vi "To Serial Form.vi"(6 "Serial Version":T1, 10 "Serializer in":refnum<class "Serializer.lvclass">, 11 "CRDS Cell in":refnum<class "CRDS Cell.lvclass">) -> (0 "error out":errorcluster, 2 "Serializer out":refnum<class "Serializer.lvclass">, 3 "CRDS Cell out":refnum<class "CRDS Cell.lvclass">)   [LabVIEW 2012, in "CRDS Cell.lvclass"]
uses:
  CRDS Cell.lvclass
  <userlib>/Serialization/Serializer/Serializer.lvclass
  <userlib>/Serialization/Serialization Common/Serial Version.ctl
  <userlib>/Serialization/Serializable/Serializable.lvclass
  CRDS Cell.lvclass/CRDS Cell.ctl
  Get Tau Method.ctl
  <userlib>/Serialization/Serializer/Serializer.lvclass/Serializer.ctl
  <userlib>/Serialization/Formatter/Formatter.lvclass/Formatter.ctl
  <userlib>/Serialization/Serializable/Insert Double.vi
  <userlib>/Serialization/Serializable/Insert Single.vi
  <userlib>/Serialization/Serializable/Insert Int08.vi
  <userlib>/Serialization/Serializable/Insert Boolean.vi
  <userlib>/Serialization/Serializable/Insert UInt08.vi
  <userlib>/Serialization/Serializer/Insert Double.vi
  <userlib>/Serialization/Serializer/Insert Single.vi
  <userlib>/Serialization/Serializer/Insert Int08.vi
  <userlib>/Serialization/Serializer/Insert Boolean.vi
  <userlib>/Serialization/Serializer/Insert UInt08.vi
  <userlib>/Serialization/Formatter/Read Include all fields.vi
  <userlib>/Serialization/Serialization Common/Serialization Common.lvlib
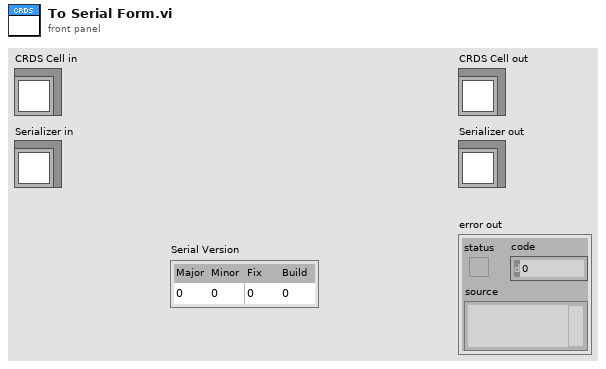
[diagram p1: front panel]
types:
  T1 = typedef "Serialization Common.lvlib/Serial Version.ctl" = cluster{"Major":u16, "Minor":u16, "Fix":u16, "Build":u16}
  T2 = typedef "Get Tau Method.ctl" = enum8{"DFT-1", "DFT-5", "LRS"}
  T3 = cluster{"inSeriesPos":u8, "numInBank":u8, "totNum":u8}
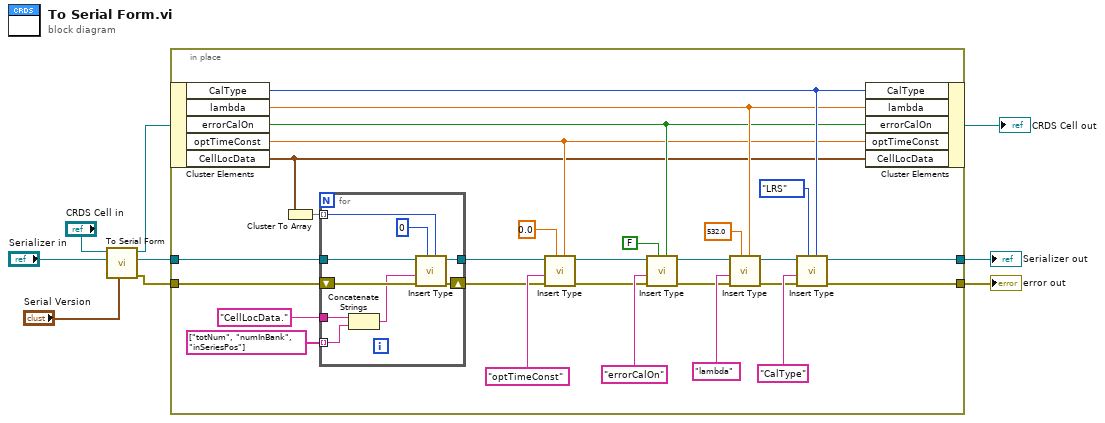
[diagram p0: block diagram]
diagram:
  n1 = call-parent "To Serial Form.vi"("Serial Version"="Serial Version", "Serializer in"="Serializer in", "Serializable in"="CRDS Cell in") -> ("error out"=w2:errorcluster, "Serializer out"=w5:refnum<class "Serializer.lvclass">, "Serializable out"=w6:refnum<class "CRDS Cell.lvclass">)  [unwired: 6 in]
  n2 = in-place {
    in-place-border: w5 -> [w11]
    in-place-border: [w29] -> w3
    in-place-border: w2 -> [w10]
    in-place-border: [w24] -> w1
    n3 = in-place-cluster #1(w6) -> ("CalType"=w19:T2, "lambda"=w18:dbl, "errorCalOn"=w17:bool, "optTimeConst"=w16:sgl, "CellLocData"=w15:T3)
    n4 = Cluster To Array(cluster=w15) -> (array=w12:u8[])
    n5 = for {
      tunnel: w11 -> [w46]
      tunnel: [w45] -> w33
      shift-right: [w43] -> w28
      shift-left: w10 -> [w44]
      tunnel: string[] ["totNum", "numInBank", "inSeriesPos"] -> [w41] mode=indexing
      tunnel: "CellLocData." ("Name") -> [w40]
      tunnel: w12 -> [w39] mode=indexing
      n6 = Concatenate Strings(w40, w41) -> (w38:string)
      n7 = call-poly <userlib>:"Insert Type.vi"("Integer"=w39, "Default Value"=u8 0, "error in (no error)"=w44, "Name"=w38, "Serializer in"=w46) -> ("error out"=w43:errorcluster, "Serializer out"=w45:refnum<class "Serializer.lvclass">)  [unwired: 5 in]
    }
    n8 = call-poly <userlib>:"Insert Type.vi"("Double"=w16, "Default Value"=sgl 0.0, "error in (no error)"=w28, "Name"="optTimeConst", "Serializer in"=w33) -> ("error out"=w27:errorcluster, "Serializer out"=w32:refnum<class "Serializer.lvclass">)  [unwired: 5 in]
    n9 = call-poly <userlib>:"Insert Type.vi"("Boolean"=w17, "Default Value"=FALSE, "error in (no error)"=w27, "Name"="errorCalOn", "Serializer in"=w32) -> ("error out"=w26:errorcluster, "Serializer out"=w31:refnum<class "Serializer.lvclass">)  [unwired: 5 in]
    n10 = call-poly <userlib>:"Insert Type.vi"("Double"=w18, "Default Value"=532.0, "error in (no error)"=w26, "Name"="lambda", "Serializer in"=w31) -> ("error out"=w25:errorcluster, "Serializer out"=w30:refnum<class "Serializer.lvclass">)  [unwired: 5 in]
    n11 = call-poly <userlib>:"Insert Type.vi"("Integer"=w19, "Default Value"=Get_Tau_Method."LRS" ("CalType"), "error in (no error)"=w25, "Name"="CalType", "Serializer in"=w30) -> ("error out"=w24:errorcluster, "Serializer out"=w29:refnum<class "Serializer.lvclass">)  [unwired: 5 in]
    n12 = in-place-cluster #1("CalType"=w19, "lambda"=w18, "errorCalOn"=w17, "optTimeConst"=w16, "CellLocData"=w15) -> (→"CRDS Cell out":refnum<class "CRDS Cell.lvclass">)
  }
  "error out" <- w1
  "Serializer out" <- w3
